vi "System Closing.vi"() -> ()   [LabVIEW 2020]
uses:
  CCD Project/Subroutines/Parameters#2.ctl
  CCD Project/Subroutines/Parameters#1.ctl
  CCD Project/Subroutines/Parameters_Control.ctl
panel:
  out "Saving Done?":bool=TRUE
  in  "Current Path":path=path "/DATA"
  in  "Control Parameters":T1={"Grating Density"=enum."1200", "Offset"=0.0, "Save All Data in ONE file"=FALSE, "Auto Save Data"=FALSE, "Most recent saved file"=path "erererere", "Filename Prefix"="MyData", "Extension"=4, "Suffix"="", "Current Path"=path "/DATA"} {"Extension" items=["DOS field", "\".001\",\".002\", ...", "001 (No dot)", "\".A\",\".B\", ...", "±Field", "pField nField", "Temperature", "User Defined"]; "Offset" format="%.2f"}
  in  "Parameters":T2={"Magnetic Field"=0.0, "Temperature"=0.0, "Exposure Time"=0.0, "Mag ID string"="Cell 12", "User Name"="Albert Einstein", "Comments"="", "SaveComments?"=1, "X-Axis Unit"=1, "Delimiter"=0, "File Format"=0, "Sample Name"="Sample1"} {"File Format" items=["Macintosh (EOL: CR)", "Unix (EOL: LF)", "DOS/Windows (EOL: CR+LF)"]; "Delimiter" items=["TAB", "COMMA", "SPACE"]; "X-Axis Unit" items=["Point #", "nm", "eV", "meV", "cm-1"]; "SaveComments?" items=["Bare data only", "Saved in the Header Area", "Saved as a Parameter File"]; "Exposure Time" format="%.2f"; "Temperature" format="%.2f"; "Magnetic Field" format="%.2f"}
  in  "Suffix":string
  in  "Background":i32[](array[numeric])=[1198, 1190, 1193, 1194, 1189, 1188, 1196, 1190, 1202, 1191, 1193, 1192, 1199, 1189, 1194, 1189, 1197, 1191, 1187, 1192, 1195, 1189, 1195, 1191, 1199, 1194, 1192, 1191, 1193, 1197, 1193, 1193, 1194, 1200, 1191, 1190, 1187, 1195, 1189, 1188, 1191, 1194, 1187, 1192, 1198, 1193, 1190, 1192, 1190, 1193, 1191, 1190, 1191, 1189, 1192, 1194, 1190, 1193, 1193, 1191, 1194, 1182, 1190, 1188, 1199, 1192, 1196, 1195, 1186, 1189, 1188, 1185, 1194, 1187, 1193, 1194, 1190, 1189, 1189, 1187, 1196, 1195, 1191, 1197, 1192, 1200, 1187, 1194, 1189, 1193, 1195, 1196, 1186, 1192, 1190, 1194, 1194, 1190, 1191, 1193, 1197, 1197, 1185, 1199, 1190, 1195, 1196, 1184, 1193, 1193, 1193, 1191, 1189, 1190, 1199, 1193, 1191, 1194, 1191, 1192, 1186, 1190, 1194, 1189, 1194, 1190, 1191, 1192, 1192, 1196, 1192, 1192, 1189, 1193, 1198, 1186, 1191, 1193, 1187, 1194, 1190, 1190, 1191, 1189, 1194, 1195, 1189, 1192, 1185, 1193, 1192, 1192, 1189, 1191, 1191, 1190, 1196, 1194, 1193, 1191, 1189, 1191, 1196, 1192, 1192, 1189, 1196, 1191, 1193, 1192, 1188, 1190, 1194, 1192, 1185, 1191, 1194, 1191, 1189, 1195, 1192, 1196, 1190, 1193, 1191, 1189, 1194, 1195, 1191, 1187, 1190, 1196, 1196, 1192, 1197, 1191, 1189, 1192, 1192, 1200, 1192, 1193, 1190, 1192, 1187, 1198, 1186, 1196, 1201, 1199, 1200, 1191, 1196, 1200, 1192, 1191, 1193, 1185, 1192, 1194, 1186, 1190, 1188, 1189, 1201, 1197, 1191, 1194, 1193, 1194, 1195, 1198, 1200, 1192, 1192, 1193, 1193, 1195, 1187, 1193, 1192, 1187, 1189, 1186, 1191, 1197, 1191, 1200, 1194, 1192, 1187, 1196, 1191, 1191, 1196, 1187, 1190, 1193, 1189, 1193, 1190, 1188, 1188, 1190, 1197, 1188, 1191, 1195, 1188, 1191, 1188, 1194, 1193, 1187, 1200, 1192, 1197, 1190, 1196, 1200, 1191, 1189, 1193, 1189, 1186, 1196, 1185, 1198, 1195, 1186, 1191, 1197, 1191, 1193, 1195, 1193, 1191, 1198, 1189, 1183, 1200, 1197, 1192, 1192, 1192, 1196, 1191, 1190, 1194, 1188, 1198, 1193, 1195, 1190, 1187, 1192, 1191, 1195, 1188, 1190, 1191, 1187, 1189, 1185, 1189, 1196, 1198, 1191, 1190, 1196, 1197, 1193, 1187, 1186, 1195, 1191, 1193, 1192, 1196, 1190, 1192, 1192, 1192, 1190, 1195, 1192, 1191, 1193, 1197, 1184, 1190, 1188, 1192, 1194, 1190, 1193, 1195, 1195, 1194, 1189, 1193, 1191, 1194, 1186, 1189, 1192, 1191, 1182, 1190, 1197, 1194, 1188, 1193, 1191, 1186, 1194, 1197, 1193, 1191, 1187, 1194, 1194, 1191, 1189, 1195, 1194, 1189, 1196, 1187, 1186, 1192, 1194, 1196, 1191, 1193, 1191, 1188, 1190, 1199, 1198, 1196, 1196, 1190, 1194, 1191, 1194, 1187, 1195, 1190, 1194, 1196, 1194, 1189, 1193, 1189, 1194, 1189, 1195, 1192, 1194, 1193, 1191, 1197, 1187, 1189, 1189, 1188, 1197, 1192, 1189, 1193, 1194, 1183, 1202, 1187, 1192, 1184, 1188, 1186, 1193, 1189, 1195, 1189, 1193, 1197, 1189, 1194, 1191, 1194, 1192, 1191, 1191, 1196, 1194, 1190, 1193, 1192, 1195, 1197, 1198, 1193, 1202, 1196, 1194, 1194, 1190, 1193, 1190, 1195, 1192, 1187, 1194, 1197, 1190, 1194, 1189, 1198, 1192, 1191, 1192, 1192, 1191, 1191, 1193, 1191, 1191, 1198, 1186, 1192, 1185, 1185, 1188, 1194, 1196, 1194, 1195, 1190, 1194, 1191, 1190, 1195, 1191, 1191, 1195, 1192, 1194, 1201, 1187, 1191, 1195, 1187, 1192, 1192, 1193, 1200, 1188, 1189, 1189, 1197, 1189, 1188, 1197, 1195, 1191, 1189, 1190, 1195, 1189, 1191, 1194, 1186, 1192, 1190, 1191, 1188, 1195, 1192, 1191, 1191, 1199, 1190, 1190, 1190, 1192, 1187, 1193, 1197, 1197, 1186, 1193, 1189, 1192, 1197, 1184, 1187, 1188, 1192, 1192, 1192, 1189, 1192, 1190, 1194, 1191, 1186, 1196, 1194, 1189, 1193, 1191, 1186, 1189, 1193, 1195, 1196, 1197, 1199, 1194, 1190, 1193, 1194, 1190, 1198, 1196, 1194, 1195, 1194, 1184, 1188, 1195, 1197, 1190, 1194, 1190, 1191, 1195, 1198, 1188, 1193, 1194, 1195, 1198, 1195, 1191, 1197, 1192, 1198, 1190, 1196, 1191, 1194, 1188, 1189, 1198, 1192, 1198, 1195, 1185, 1191, 1193, 1192, 1197, 1195, 1195, 1195, 1193, 1190, 1190, 1190, 1198, 1195, 1191, 1194, 1190, 1190, 1194, 1194, 1195, 1192, 1190, 1194, 1195, 1192, 1192, 1194, 1189, 1192, 1193, 1188, 1194, 1195, 1196, 1193, 1192, 1201, 1191, 1198, 1197, 1191, 1192, 1191, 1194, 1193, 1188, 1192, 1189, 1183, 1189, 1190, 1192, 1189, 1196, 1193, 1197, 1185, 1193, 1189, 1191, 1196, 1195, 1193, 1193, 1191, 1189, 1193, 1192, 1192, 1192, 1190, 1191, 1193, 1193, 1197, 1195, 1189, 1193, 1188, 1194, 1197, 1194, 1195, 1196, 1190, 1194, 1188, 1197, 1195, 1191, 1195, 1192, 1194, 1188, 1190, 1197, 1197, 1191, 1187, 1197, 1191, 1193, 1188, 1191, 1194, 1193, 1195, 1192, 1195, 1189, 1193, 1193, 1195, 1190, 1192, 1196, 1188, 1187, 1193, 1192, 1192, 1194, 1185, 1199, 1190, 1193, 1191, 1198, 1189, 1190, 1191, 1190, 1193, 1195, 1186, 1190, 1193, 1191, 1189, 1197, 1193, 1198, 1190, 1192, 1193, 1191, 1196, 1193, 1196, 1190, 1190, 1198, 1192, 1199, 1198, 1190, 1191, 1191, 1196, 1190, 1196, 1195, 1191, 1196, 1195, 1193, 1190, 1190, 1195, 1193, 1187, 1197, 1185, 1191, 1189, 1191, 1193, 1192, 1188, 1196, 1193, 1191, 1193, 1193, 1190, 1192, 1192, 1192, 1195, 1191, 1195, 1189, 1189, 1191, 1191, 1185, 1192, 1191, 1193, 1201, 1199, 1197, 1206, 1201, 1207, 1200, 1198, 1195, 1188, 1194, 1186, 1190, 1197, 1188, 1193, 1196, 1193, 1192, 1192, 1188, 1196, 1186, 1193, 1194, 1188, 1190, 1190, 1192, 1190, 1191, 1191, 1200, 1192, 1199, 1193, 1190, 1190, 1199, 1187, 1193, 1190, 1188, 1194, 1194, 1196, 1194, 1195, 1190, 1187, 1187, 1196, 1193, 1199, 1190, 1193, 1193, 1191, 1198, 1192, 1193, 1192, 1193, 1189, 1189, 1197, 1189, 1194, 1193, 1192, 1185, 1198, 1193, 1189, 1192, 1193, 1196, 1190, 1195, 1189, 1196, 1198, 1190, 1191, 1193, 1186, 1189, 1195, 1188, 1197, 1188, 1191, 1185, 1190, 1193, 1188, 1198, 1192, 1193, 1194, 1194, 1189, 1184, 1193, 1199, 1193, 1192, 1193, 1190, 1196, 1191, 1192, 1189, 1194, 1188, 1189, 1190, 1190, 1192, 1195, 1188, 1190, 1192, 1189, 1197, 1192, 1194, 1187, 1196, 1192, 1194, 1185, 1187, 1187, 1191, 1195, 1190, 1186, 1183, 1194, 1194, 1192, 1192, 1188, 1193, 1195, 1189, 1190, 1191, 1192, 1196, 1186, 1195, 1191, 1185, 1191, 1187, 1190, 1188, 1189, 1187, 1196, 1191, 1190, 1191, 1190, 1196, 1195, 1186, 1187, 1187, 1188, 1194, 1192, 1192, 1192, 1189, 1192, 1191, 1188, 1188, 1187, 1187, 1190, 1186, 1191, 1195, 1192, 1196, 1193, 1192, 1191, 1189, 1187, 1193, 1188, 1189, 1194, 1191, 1185, 1193, 1191, 1196, 1196, 1199, 1195, 1211]
  in  "Offset":dbl format="%.2f"
  in  "FieldRamp Parameters":dbl[][](array[numeric])=[[0.0, 30.0, 1.0, 400.0], [30.0, 0.0, -1.0, 400.0], [0.0, -30.0, -1.0, 400.0], [-30.0, 0.0, 1.0, 400.0], [0.0, 30.0, 0.5, 200.0], [30.0, 0.0, -0.5, 200.0]] step=1.0 format="%.2f"
  in  "Auto Save Data":bool caption="Manual"
  out "Most recent saved file":path=path "erererere"
  in  "Filename Prefix":string="MyData"
  in  "Extension":u16(ring)=4 items=["DOS field", "\".001\",\".002\", ...", "001 (No dot)", "\".A\",\".B\", ...", "±Field", "pField nField", "Temperature", "User Defined"]
  in  "X-Axis Array":dbl[][](array[numeric])=array1025x10[10250 elements] format="%.2f"
  in  "Data Array":dbl[][](array[numeric])=array1025x10[10250 elements] format="%.2f"
  out "Parameters#2":T3={"MaxBufferSize"=2, "Mag GPIB Address"=5, "Max Current (kA)"=36.0, "LTC-GPIB Address"="", "Temp Tolerance"=1.0} {"Temp Tolerance" format="%.2f"; "Max Current (kA)" format="%.2f"}
  out "ExperimentStatus":string
  in  "Quit":bool
  in  "Save All Data in ONE file":bool caption="Save in MULTIPLE files"
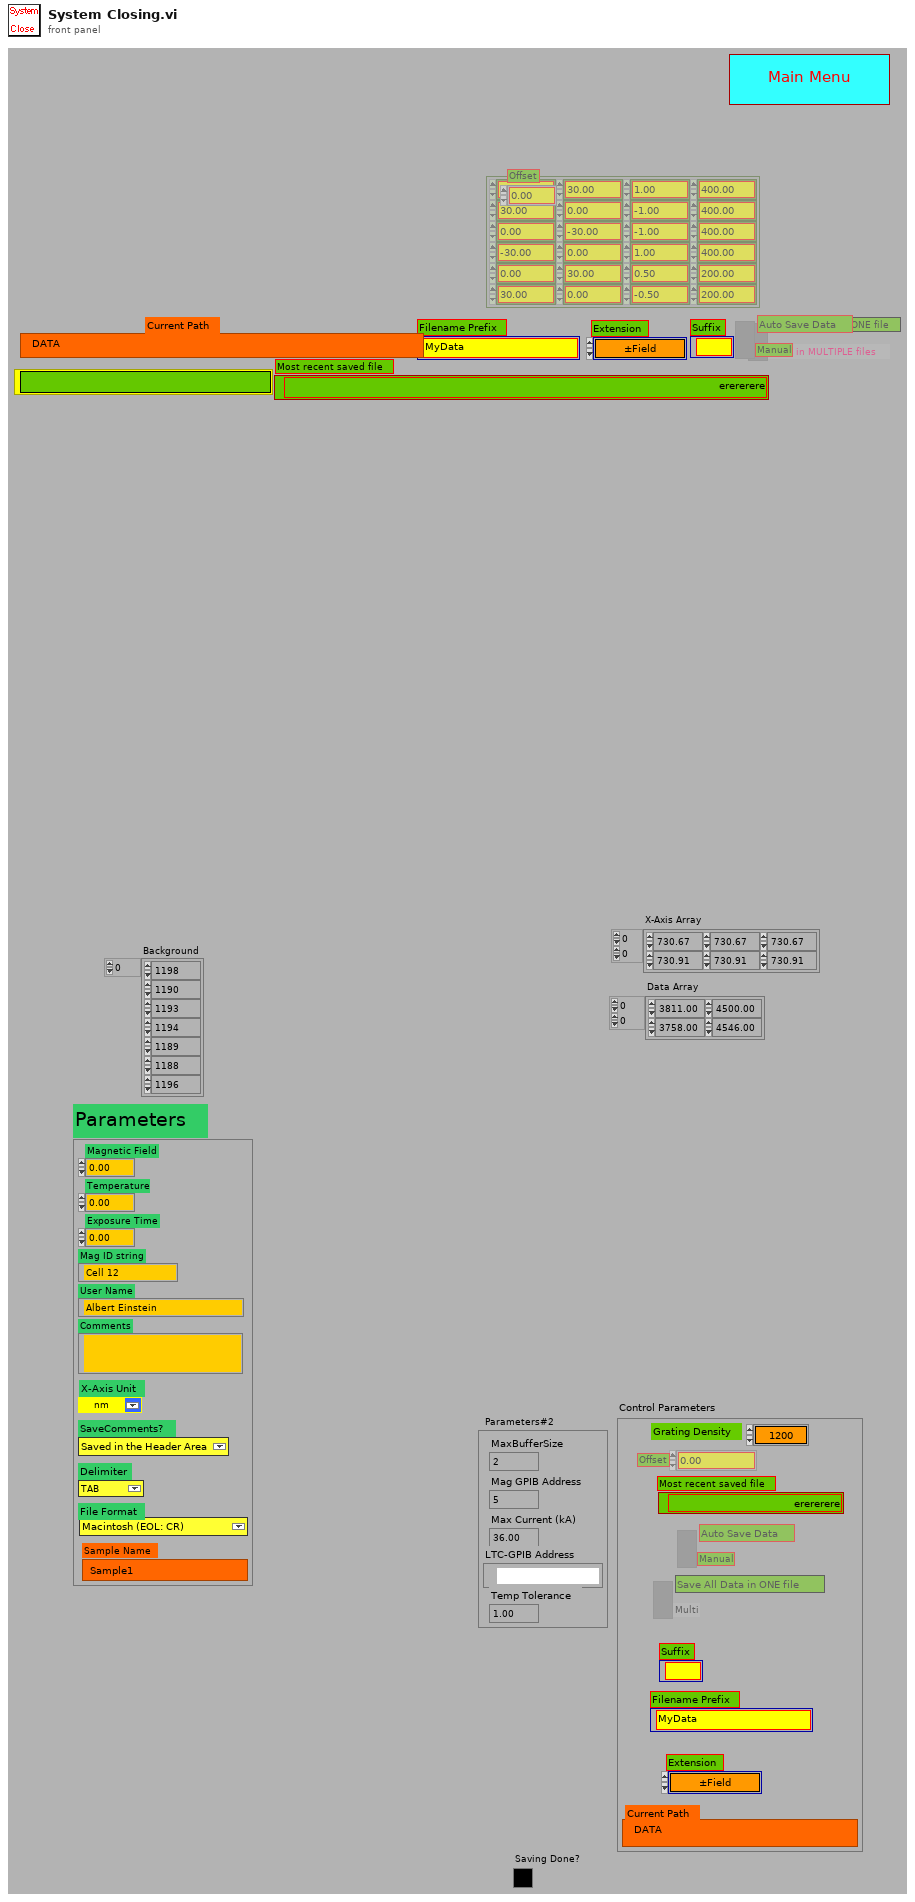
[diagram p1: front panel]
types:
  T1 = typedef "Parameters_Control.ctl" = cluster{"Grating Density":enum16{"150", "300", "600", "1200", "1800"}, "Offset":dbl, "Save All Data in ONE file":bool, "Auto Save Data":bool, "Most recent saved file":path, "Filename Prefix":string, "Extension":u16, "Suffix":string, "Current Path":path}
  T2 = typedef "Parameters#1.ctl" = cluster{"Magnetic Field":dbl, "Temperature":dbl, "Exposure Time":dbl, "Mag ID string":string, "User Name":string, "Comments":string, "SaveComments?":u16, "X-Axis Unit":u16, "Delimiter":u16, "File Format":u16, "Sample Name":string}
  T3 = typedef "Parameters#2.ctl" = cluster{"MaxBufferSize":i32, "Mag GPIB Address":i32, "Max Current (kA)":dbl, "LTC-GPIB Address":refnum<visa-resource-name>, "Temp Tolerance":dbl}
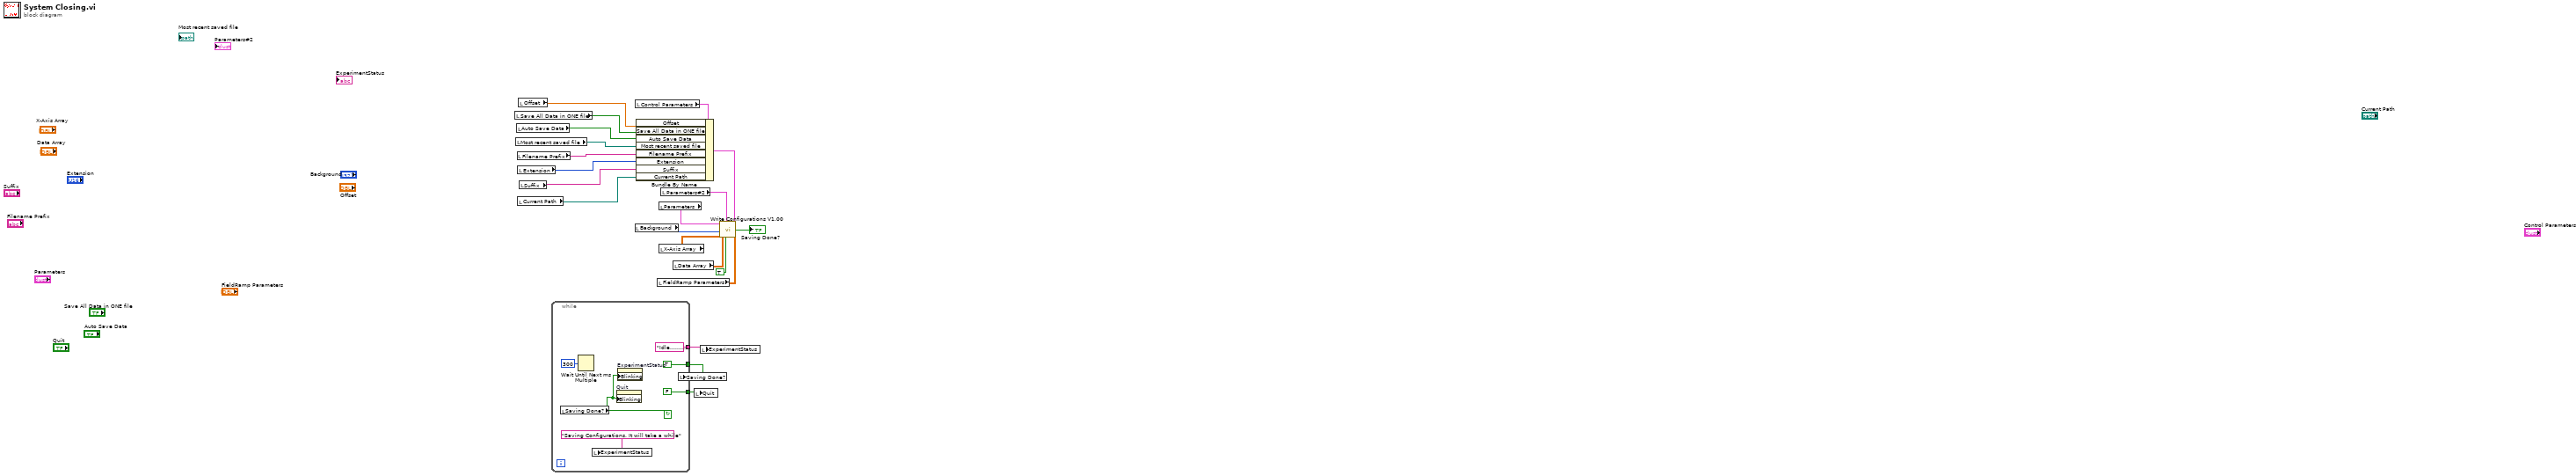
[diagram p0: block diagram]
diagram:
  n1 = local read "Save All Data in ONE file"() -> (w19:bool)
  n2 = local read "Most recent saved file"() -> (w17:path)
  n3 = local read "Auto Save Data"() -> (w18:bool)
  n4 = local read "Filename Prefix"() -> (w16:string)
  n5 = local read "Extension"() -> (w15:u16)
  n6 = local read "Current Path"() -> (w13:path)
  n7 = local read "Offset"() -> (w20:dbl)
  n8 = local read "Suffix"() -> (w14:string)
  n9 = while {
    tunnel: [TRUE] -> w2
    tunnel: ["Idle........."] -> w3
    tunnel: [FALSE] -> w4
    stop <- w23 continue-if-true
    n10 = local read "Saving Done?"() -> (w23:bool)
    n11 = Wait Until Next ms Multiple(millisecond multiple=u32 300) -> ()  [unwired: 1 out]
    n12 = local write "ExperimentStatus"("Saving Configurations. It will take a while" ("ExperimentStatus")) -> ()
    n13 = property on="Quit" class="Bool (strict)"("Blinking"=w23) -> ()  [unwired: 2 in, 2 out]
    n14 = property on="ExperimentStatus" class="Str"("Blinking"=w23) -> ()  [unwired: 2 in, 2 out]
  }
  n15 = local read "Background"() -> (w9:i32[])
  n16 = local read "Control Parameters"() -> (w21:T1)
  n17 = Bundle By Name(cluster=w21, "Offset"=w20, "Save All Data in ONE file"=w19, "Auto Save Data"=w18, "Most recent saved file"=w17, "Filename Prefix"=w16, "Extension"=w15, "Suffix"=w14, "Current Path"=w13) -> (w10:T1)
  n18 = local read "FieldRamp Parameters"() -> (w6:dbl[][])
  n19 = local read "Parameters"() -> (w12:T2)
  n20 = local read "X-Axis Array"() -> (w8:dbl[][])
  n21 = local read "Parameters#2"() -> (w11:T3)
  n22 = local read "Data Array"() -> (w7:dbl[][])
  n23 = local write "Saving Done?"(w2) -> ()
  n24 = local write "Quit"(w4) -> ()
  n25 = local write "ExperimentStatus"(w3) -> ()
  n26 = call "Write Configurations V1.00.vi"("FieldRamp Parameters"=w6, "Control Parameters"=w10, "SaveParameters(T)/DataBuffer(F)?"=TRUE ("SaveParametersOnly?"), "Parameters#2"=w11, "X-Axis Array"=w8, "Background"=w9, "Data Array"=w7, "Parameters"=w12) -> ("Done"=→"Saving Done?":bool)  [unwired: 2 in]
